vi "SearchEnumProcessInSetup.vi"(8 "error in (no error)":errorcluster, 10 "FlatSequenceFrame in":refnum<vi>, 11 "AppContextIn":T1={"VIRefToProcessTemplate"=refnum, "VIRefToThisVI"=refnum, "ProcessesList"=[], "VIRefToEnumProcess"=refnum, "VIRefTogetProcessViPath"=refnum, "ProcessManagement"={"EnumProcessState"=enum."Create process", "ProcessName"="", "PathToProcess"=path ""}, "VIRefToSetup"=refnum, "VIRefToStartProcess"=refnum, "ProcessConfig"={"File Path Control"=path "", "Timeout"=0.0, "viInitString"="", "State"=enum."Closed"}}) -> (0 "error out":errorcluster, 2 "EnumConstant out":refnum<vi>, 3 "AppContextOut":T1={"VIRefToProcessTemplate"=refnum, "VIRefToThisVI"=refnum, "ProcessesList"=[], "VIRefToEnumProcess"=refnum, "VIRefTogetProcessViPath"=refnum, "ProcessManagement"={"EnumProcessState"=enum."Create process", "ProcessName"="", "PathToProcess"=path ""}, "VIRefToSetup"=refnum, "VIRefToStartProcess"=refnum, "ProcessConfig"={"File Path Control"=path "", "Timeout"=0.0, "viInitString"="", "State"=enum."Closed"}})   [LabVIEW 2011]
uses:
  Ctl/AppContext.ctl
  Ctl/EnumProcessState.ctl
  050 - CONFIG/20 - ExternalProcesses/paramsExternalProcesses.ctl
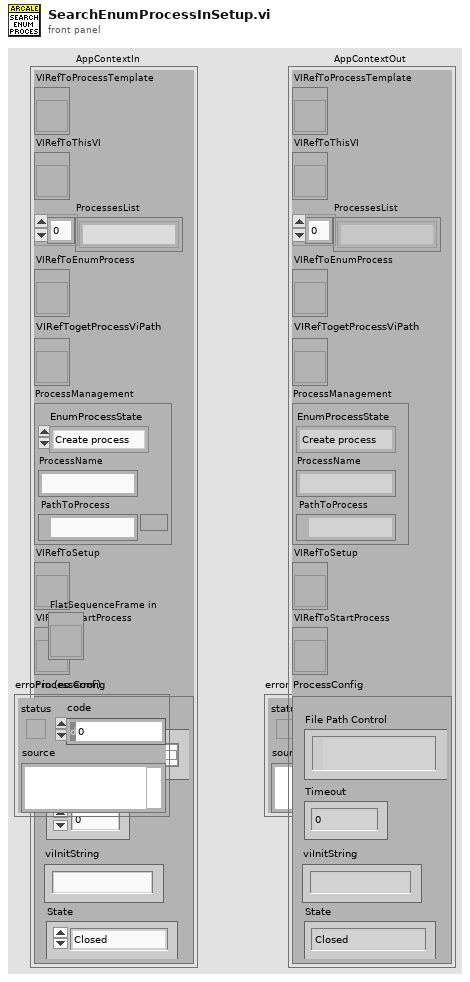
[diagram p1: front panel]
types:
  T1 = typedef "AppContext.ctl" = cluster{"VIRefToProcessTemplate":refnum<vi>, "VIRefToThisVI":refnum<vi>, "ProcessesList":string[], "VIRefToEnumProcess":refnum<vi>, "VIRefTogetProcessViPath":refnum<vi>, "ProcessManagement":cluster{"EnumProcessState":T2, "ProcessName":string, "PathToProcess":path}, "VIRefToSetup":refnum<vi>, "VIRefToStartProcess":refnum<vi>, "ProcessConfig":T3}
  T2 = typedef "EnumProcessState.ctl" = enum16{"Create process", "Delete process"}
  T3 = typedef "paramsExternalProcesses.ctl" = cluster{"File Path Control":path, "Timeout":dbl, "viInitString":string, "State":enum32{"Invalid", "Standard", "Closed", "Hidden", "Minimized", "Maximized"}}
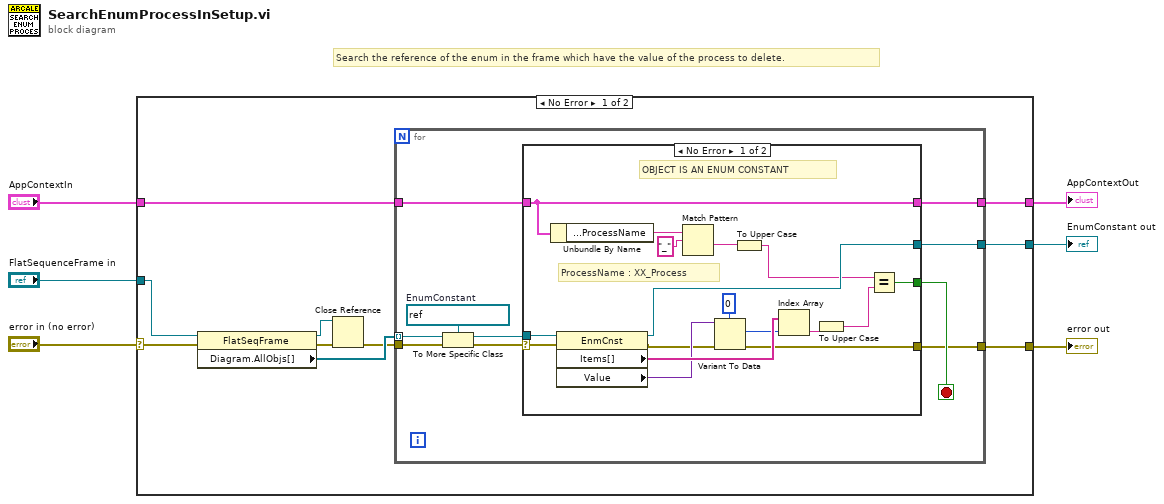
[diagram p0: block diagram]
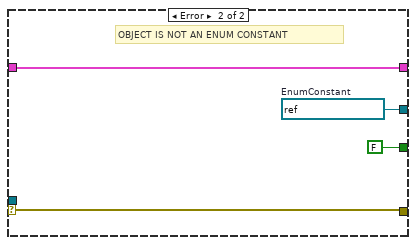
[diagram p2: hidden frame]
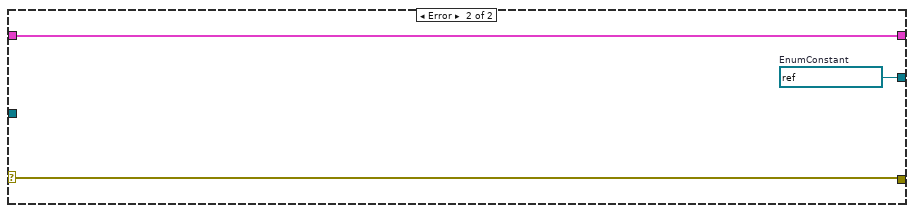
[diagram p3: hidden frame]
diagram:
  # "Search the reference of the enum in the frame which have the value of the process to delete."
  n1 = case shown="No Error" "error in (no error)" {
    selector: "error in (no error)" -> [w12 w50]
    tunnel: [w16 w49] -> w6
    tunnel: "AppContextIn" -> [w15 w48]
    tunnel: "FlatSequenceFrame in" -> [w13 _]
    tunnel: [w11 w50] -> w2
    tunnel: [w10 w48] -> w1
    frame No Error {
      n2 = property class="FlatSeqFrame"(reference=w13, error in=w12) -> (reference out=w9:refnum<vi>, error out=w8:errorcluster, "Diagram.AllObjs[]"=w14:refnum<vi>[])
      n3 = Close Reference(reference=w9, error in (no error)=w8) -> (error out=w7:errorcluster)
      n4 = for {
        tunnel: w14 -> [w17] mode=indexing
        tunnel: w7 -> [w25]
        tunnel: w15 -> [w22]
        tunnel: [w20] -> w16
        tunnel: [w19] -> w11
        tunnel: [w18] -> w10
        stop <- w21 stop-if-true
        w26 = refnum<vi> refnum  # EnumConstant
        n5 = To More Specific Class(target class=w26, reference=w17, error in=w25) -> (specific class reference=w23:refnum<vi>, error out=w24:errorcluster)
        n6 = case shown="No Error" w24 {
          selector: w24 -> [w36 w45]
          tunnel: w23 -> [w43 _]
          tunnel: w22 -> [w33 w44]
          tunnel: [w38 FALSE] -> w21
          tunnel: [w37 w46] -> w20
          tunnel: [w34 w45] -> w19
          tunnel: [w33 w44] -> w18
          frame No Error {
            # "ProcessName : XX_Process"
            # "OBJECT IS AN ENUM CONSTANT"
            n7 = Unbundle By Name(w33) -> ("ProcessManagement.ProcessName"=w31:string)
            n8 = property class="EnmCnst"(reference=w43, error in=w36) -> (reference out=w37:refnum<vi>, error out=w35:errorcluster, "Items[]"=w42:string[], "Value"=w41:variant)
            n9 = Match Pattern(string=w31, regular expression="_") -> (after substring=w27:string)  [unwired: 1 in, 3 out]
            n10 = Variant To Data(error in=w35, type=0, Variant=w41) -> (data=w39:i32, error out=w34:errorcluster)
            n11 = To Upper Case(1:w27) -> (0:w30:string)
            n12 = Index Array(array=w42, index=w39) -> (element=w29:string)
            n13 = To Upper Case(1:w29) -> (0:w28:string)
            n14 = Equal?(x=w30, y=w28) -> (x = y?=w38:bool)
          }
          frame Error {
            w46 = refnum<vi> refnum  # EnumConstant
            # "OBJECT IS NOT AN ENUM CONSTANT"
          }
        }
      }
    }
    frame Error {
      w49 = refnum<vi> refnum  # EnumConstant
    }
  }
  "error out" <- w2
  "EnumConstant out" <- w6
  "AppContextOut" <- w1
